vi "Main Page.vi"(8 "error in (no error)":errorcluster, 11 "Node Ptr":T2 format="%.0x") -> (0 "error out":errorcluster)   [LabVIEW 2019, in "Instrument Addon System Explorer.lvlib"]
uses:
  Instrument Addon System Explorer.lvlib
  <vilib>/NI VeriStand/Custom Device API/Custom Device Item Ref.ctl
  Addon Shared/Types/FG Control.ctl
  <vilib>/NI/NI VeriStand Hardware Resource Discovery/_Types/Filter Type.ctl
  Addon Shared/Constants.vi
  <vilib>/NI VeriStand/Custom Device API/NI VeriStand - Get Item Property.vi
  <vilib>/NI VeriStand/Custom Device API/Get Item Property (U32).vi
  <vilib>/NI VeriStand/Custom Device API/NI VeriStand - Set Item Property.vi
  <vilib>/NI VeriStand/Custom Device API/Set Item Property (U32).vi
  <vilib>/NI VeriStand/Custom Device API/Get Item Property (String).vi
  <vilib>/NI VeriStand/Custom Device API/Set Item Property (String).vi
  <vilib>/NI VeriStand/Custom Device API/Get Item Property (Boolean).vi
  <vilib>/NI VeriStand/Custom Device API/Set Item Property (Boolean).vi
  <vilib>/Utility/LVClass/Get LV Class Default Value.vi
  Support Libraries/Protocols/Protocols.lvlibp/Protocol Parent/Protocol Parent.lvclass
  <vilib>/NI VeriStand/Custom Device API/Custom Device API.lvlib
  Addon Shared/Instrument Addon Shared.lvlib
  <vilib>/NI/NI VeriStand Hardware Resource Discovery/NIVS Hardware Discovery.lvlib
panel:
  out "Version":string
  in  "PCL Decimation":u32=1 min=1 max=10000 step=1
  in  "Protocol Settings":enum32{"RS232", "VISA", "TCP/IP", "UDP"}(tab)=enum."VISA"
  in  "COM Browse":bool
  in  "Termination Character":u8=10 format="%.0x"
  in  "End Write":bool=TRUE caption="End Write on Termination Character?"
  in  "End Read":bool=TRUE caption="End Read on Termination Character?"
  in  "XOFF":T1(ring)=enum."DC3"
  in  "XON":T1(ring)=enum."DC1"
  in  "Flow Control":u16(ring) items=["None"=0, "XON/XOFF"=1, "RTS/CTS"=2, "DTR/DSR"=4]
  in  "Stop Bits":u16(ring)=10 items=["1.0"=10, "1.5"=15, "2.0"=20]
  in  "Parity":enum16{"None", "Odd", "Even", "Mark", "Space"}(ring)
  in  "Data Bits":u16=8 min=5 max=8 step=1
  in  "Baud Rate":u32(ring)=9600 items=["75"=75, "110"=110, "134"=134, "150"=150, "300"=300, "600"=600, "1200"=1200, "1800"=1800, "2400"=2400, "4800"=4800, "7200"=7200, "9600"=9600, "14400"=14400, "19200"=19200, "28800"=28800, "38400"=38400, "56000"=56000, "57600"=57600, "115200"=115200, "128000"=128000, "230400"=230400, "460800"=460800, "921600"=921600, "1843200"=1843200, "3000000"=3000000]
  in  "Port":string="COM1"
  in  "VISA Browse":bool
  in  "Append Write Termination Character":bool caption="End Write on Termination Character?"
  in  "Timeout":u32=2000 caption="Timeout (ms)"
  in  "Termination Character":u8=10 format="%.0x"
  in  "Enable Termination Character":bool=TRUE caption="Enable Termination Character?"
  in  "VISA Resource":string="GPIB0::2::INSTR"
  in  "Port":u16
  in  "IP Address":string="localhost"
  in  "UDP Browse":bool
  in  "Target Port":u16
  in  "Target IP Address":string="localhost"
  in  "Local Port":u16
  in  "Local IP Address":string="localhost"
  in  "Protocol":string(combo)
  in  "SHDocVw.IWebBrowser":refnum<k7>(container)
  in  "Header":cluster{"Section Name":string}={"Section Name"="Custom Device Item Settings"}
  in  "Description":string
  in  "Name":string
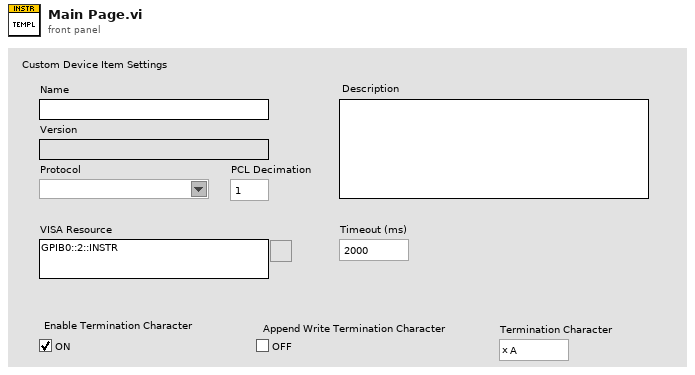
[diagram p1: front panel]
types:
  T1 = enum16{"NUL", "SOH", "STX", "ETX", "EOT", "ENQ", "ACK", "BEL", "BS", "HT", "LF", "VT", "FF", "CR", "SO", "SI", "DLE", "DC1", "DC2", "DC3", "DC4", "NAK", "SYN", "ETB", "CAN", "EM", "SUB", "ESC", "FS", "GS", "RS", "US", "SP", "!", "\"", "#", "$", "%", "&", "'", "(", ")", "*", "+", ",", "- (-)", ".", "/", "0", "1", "2", "3", "4", "5", "6", "7", "8", "9", ":", ";", "<", "=", ">", "?", "@", "A", "B", "C", "D", "E", "F", "G", "H", "I", "J", "K", "L", "M", "N", "O", "P", "Q", "R", "S", "T", "U", "V", "W", "X", "Y", "Z", "[", "\\", "]", "^", "_", "`", "a", "b", "c", "d", "e", "f", "g", "h", "i", "j", "k", "l", "m", "n", "o", "p", "q", "r", "s", "t", "u", "v", "w", "x", "y", "z", "{", "|", "}", "~"}
  T2 = typedef "Custom Device API.lvlib/Custom Device Item Ref.ctl" = u64
  T3 = typedef "Instrument Addon Shared.lvlib/FG Control.ctl" = enum16{"Get", "Set"}
  T4 = typedef "Custom Device API.lvlib/Custom Device Item Info.ctl" = cluster{"Name":string, "Is Channel":bool, "GUID":string, "Is Waveform":bool}
  T5 = typedef "NIVS Hardware Discovery.lvlib/Filter Type.ctl" = enum16{"Device Category", "Product Name", "Ethernet", "XNET", "VISA", "FPGA", "EtherCAT Master", "DAQmx", "GPIB", "Serial"}
  T6 = typedef "Custom Device API.lvlib/Custom Device Commands.ctl" = enum16{"Default", "Item renamed", "Shutdown", "Dynamic button pressed"}
  T7 = typedef "Instrument Addon Shared.lvlib/VISA Settings.ctl" = cluster{"VISA Resource":string, "Enable Termination Character":bool, "Termination Character":u8, "Timeout":u32, "Append Write Termination Character":bool}
  T8 = typedef "Instrument Addon Shared.lvlib/TCPIP Settings.ctl" = cluster{"IP Address":string, "Port":u16}
  T9 = typedef "Instrument Addon Shared.lvlib/UDP Settings.ctl" = cluster{"Local IP Address":string, "Local Port":u16, "Target IP Address":string, "Target Port":u16}
  T10 = typedef "Instrument Addon Shared.lvlib/RSXXX Port Settings.ctl" = cluster{"Port":string, "Baud Rate":u32, "Data Bits":u16, "Parity":enum16{"None", "Odd", "Even", "Mark", "Space"}, "Stop Bits":u16, "Flow Control":u16, "XON":enum16{"NUL", "SOH", "STX", "ETX", "EOT", "ENQ", "ACK", "BEL", "BS", "HT", "LF", "VT", "FF", "CR", "SO", "SI", "DLE", "DC1", "DC2", "DC3", "DC4", "NAK", "SYN", "ETB", "CAN", "EM", "SUB", "ESC", "FS", "GS", "RS", "US", "SP", "!", "\"", "#", "$", "%", "&", "'", "(", ")", "*", "+", ",", "- (-)", ".", "/", "0", "1", "2", "3", "4", "5", "6", "7", "8", "9", ":", ";", "<", "=", ">", "?", "@", "A", "B", "C", "D", "E", "F", "G", "H", "I", "J", "K", "L", "M", "N", "O", "P", "Q", "R", "S", "T", "U", "V", "W", "X", "Y", "Z", "[", "\\", "]", "^", "_", "`", "a", "b", "c", "d", "e", "f", "g", "h", "i", "j", "k", "l", "m", "n", "o", "p", "q", "r", "s", "t", "u", "v", "w", "x", "y", "z", "{", "|", "}", "~"}, "XOFF":enum16{"NUL", "SOH", "STX", "ETX", "EOT", "ENQ", "ACK", "BEL", "BS", "HT", "LF", "VT", "FF", "CR", "SO", "SI", "DLE", "DC1", "DC2", "DC3", "DC4", "NAK", "SYN", "ETB", "CAN", "EM", "SUB", "ESC", "FS", "GS", "RS", "US", "SP", "!", "\"", "#", "$", "%", "&", "'", "(", ")", "*", "+", ",", "- (-)", ".", "/", "0", "1", "2", "3", "4", "5", "6", "7", "8", "9", ":", ";", "<", "=", ">", "?", "@", "A", "B", "C", "D", "E", "F", "G", "H", "I", "J", "K", "L", "M", "N", "O", "P", "Q", "R", "S", "T", "U", "V", "W", "X", "Y", "Z", "[", "\\", "]", "^", "_", "`", "a", "b", "c", "d", "e", "f", "g", "h", "i", "j", "k", "l", "m", "n", "o", "p", "q", "r", "s", "t", "u", "v", "w", "x", "y", "z", "{", "|", "}", "~"}, "End Read on Termination Character":bool, "End Write on Termination Character":bool, "Termination Character":u8}
  T11 = typedef "Protocols.lvlibp/Protocol Parent.lvclass/Base Protocol Type.ctl" = enum16{"RS-XXX", "VISA", "TCPIP", "UDP"}
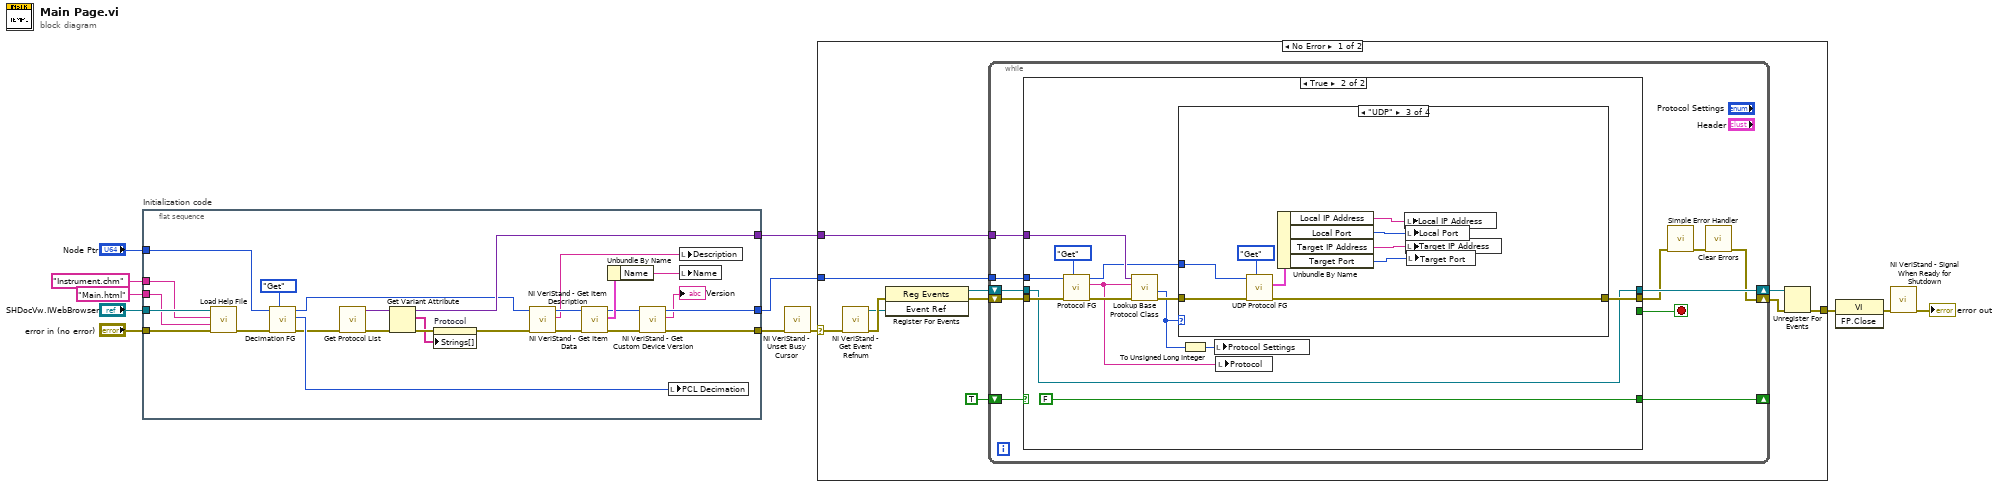
[diagram p0: block diagram]
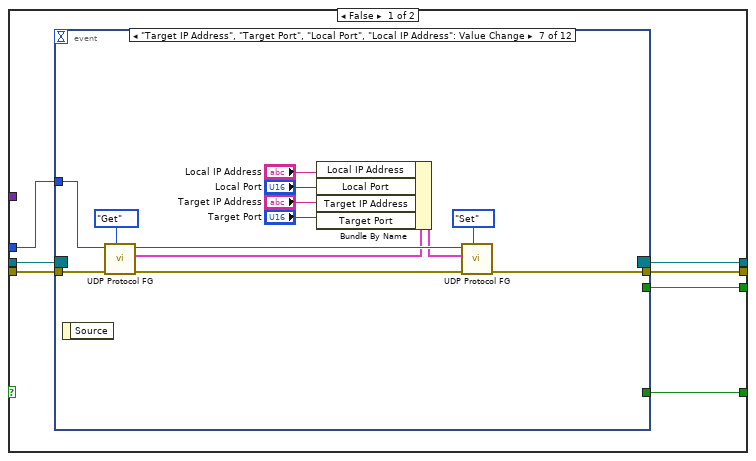
[diagram p2: hidden frame]
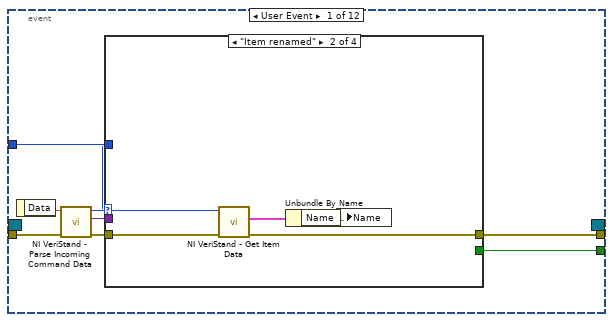
[diagram p3: hidden frame]
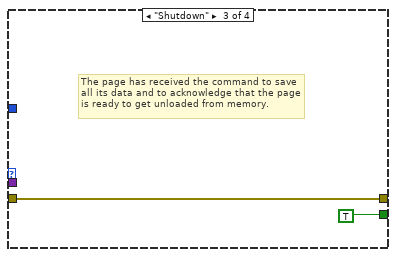
[diagram p5: hidden frame]
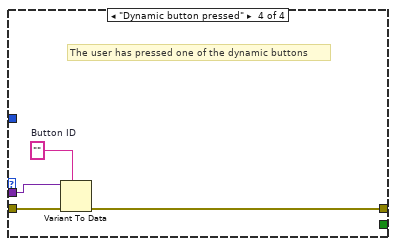
[diagram p6: hidden frame]
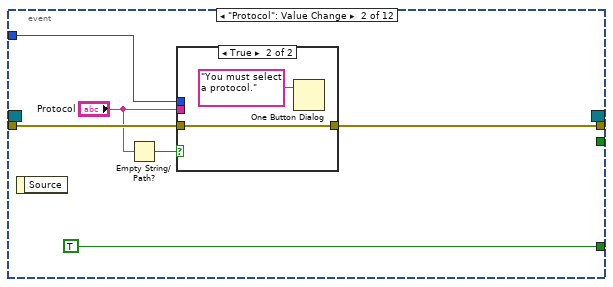
[diagram p7: hidden frame]
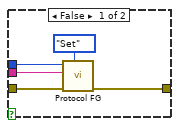
[diagram p8: hidden frame]
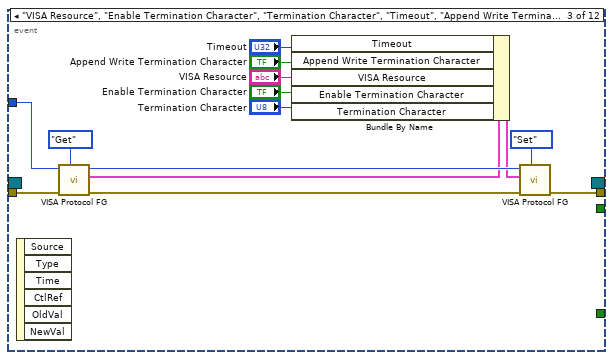
[diagram p9: hidden frame]
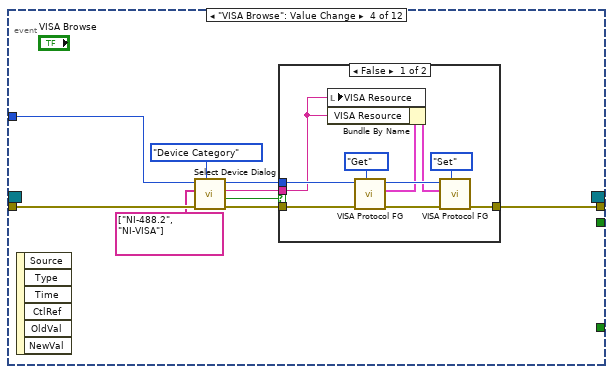
[diagram p10: hidden frame]
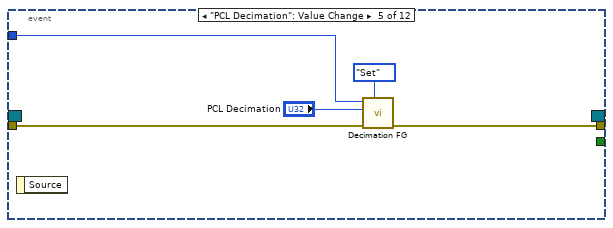
[diagram p12: hidden frame]
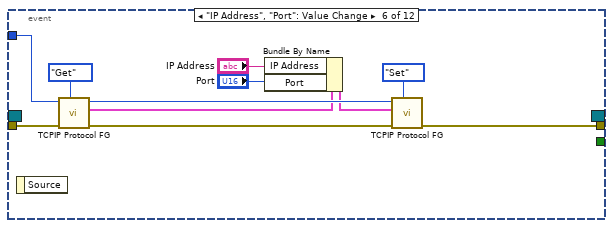
[diagram p13: hidden frame]
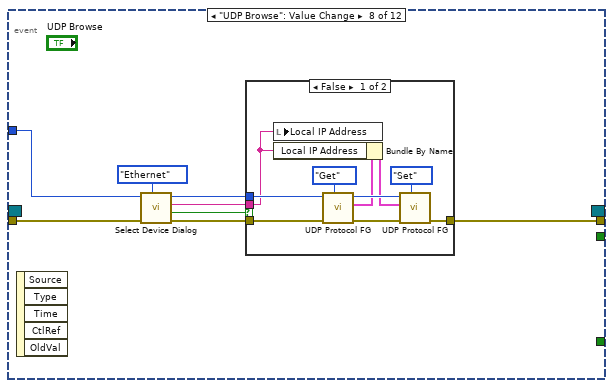
[diagram p14: hidden frame]
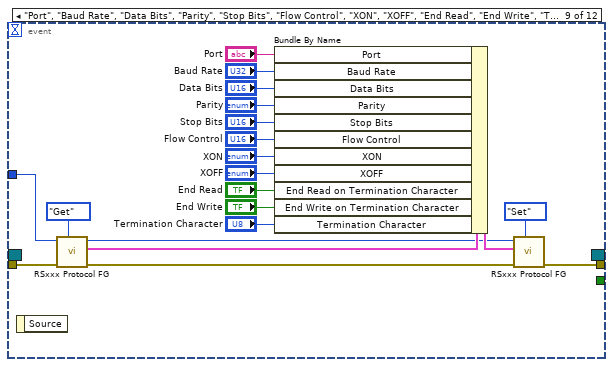
[diagram p16: hidden frame]
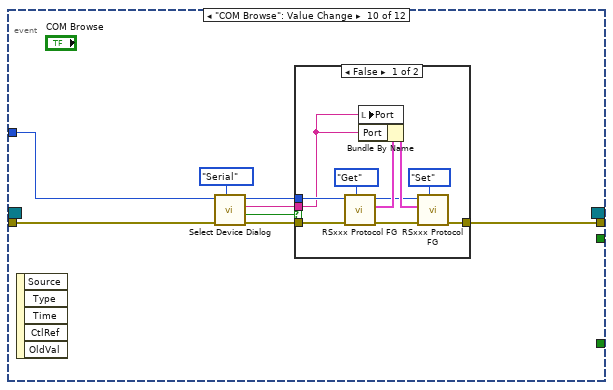
[diagram p17: hidden frame]
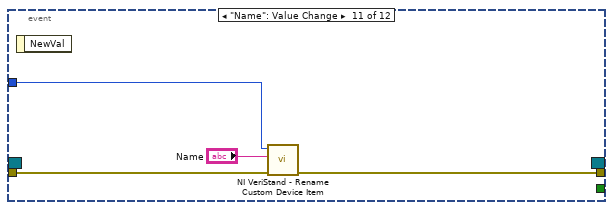
[diagram p19: hidden frame]
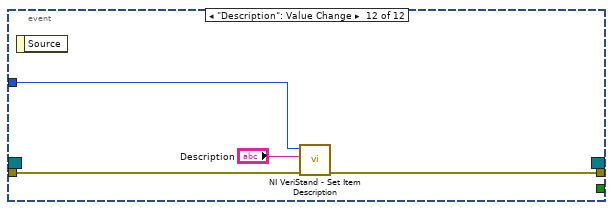
[diagram p20: hidden frame]
diagram:
  n1 = flat-sequence "Initialization code" {
    tunnel: "error in (no error)" -> [w33]
    tunnel: "Node Ptr" -> [w29]
    tunnel: [w16] -> w8
    tunnel: [w14] -> w5
    tunnel: "SHDocVw.IWebBrowser" -> [w32]
    tunnel: "Main.html" ("HTML File") -> [w31]
    tunnel: "Instrument.chm" ("Main CHM File") -> [w30]
    tunnel: [w21] -> w1
    frame #0 {
      n2 = call "Load Help File.vi"("error in (no error)"=w33, "HTML File"=w31, "Main CHM File"=w30, "SHDocVw.IWebBrowser2"=w32) -> ("error out"=w28:errorcluster)  [unwired: 7 in]
      n3 = call "Decimation FG.vi"("Action"=FG_Control."Get", "error in (no error)"=w28, "Device Item Ref in"=w29) -> ("error out"=w19:errorcluster, "Decimation out"=w26:u32, "Item Ref out"=w18:T2)  [unwired: 6 in]
      n4 = call "Get Protocol List.vi"("error in (no error)"=w19) -> ("error out"=w24:errorcluster, "Class Lookup"=w25:variant)  [unwired: 9 in]
      n5 = Get Variant Attribute(Variant=w25, error in=w24) -> (duplicate Variant=w21:variant, names=w22:string[], error out=w23:errorcluster)  [unwired: 2 in, 1 out]
      n6 = property on="Protocol" class="CmbBox"(error in=w23, "Strings[]"=w22) -> (error out=w20:errorcluster)  [unwired: 1 in, 1 out]
      n7 = call <vilib>:"NI VeriStand - Get Item Description.vi"("error in (no error)"=w20, "Item Ref in"=w18) -> ("error out"=w36:errorcluster, "Description"=w37:string, "Item Ref out"=w38:T2)  [unwired: 7 out]
      n8 = call <vilib>:"NI VeriStand - Get Item Data.vi"("error in (no error)"=w36, "Item Ref in"=w38) -> ("error out"=w17:errorcluster, "Item Info"=w35:T4, "Item Ref out"=w15:T2)  [unwired: 7 out]
      n9 = Unbundle By Name(w35) -> ("Name"=w34:string)
      n10 = call <vilib>:"NI VeriStand - Get Custom Device Version.vi"("error in (no error)"=w17, "Device Ref in"=w15) -> ("error out"=w16:errorcluster, "Value"=→"Version":string, "Device Ref out"=w14:T2)  [unwired: 7 in]
      n11 = local write "PCL Decimation"(w26) -> ()
      n12 = local write "Description"(w37) -> ()
      n13 = local write "Name"(w34) -> ()
    }
  }
  n14 = call <vilib>:"NI VeriStand - Unset Busy Cursor.vi"("error in (no error)"=w8) -> ("error out"=w7:errorcluster)  [unwired: 10 out]
  n15 = case shown="No Error" w7 {
    selector: w7 -> [w41 w287]
    tunnel: [w46 w285] -> w12
    tunnel: w5 -> [w42 _]
    tunnel: w1 -> [w40 _]
    frame No Error {
      n16 = call <vilib>:"NI VeriStand - Get Event Refnum.vi"("error in (no error)"=w41) -> ("error out"=w49:errorcluster, "Event Ref"=w45:refnum<user-event>)  [unwired: 9 out]
      n17 = register-events(error in=w49, w45) -> (reference out=w43:refnum<event-registration>, error out=w44:errorcluster)  [unwired: 1 in]
      n18 = while {
        tunnel: w42 -> [w56]
        shift-right: [w53] -> w47
        shift-left: w44 -> [w59]
        shift-right: [w60] -> w48
        shift-left: w43 -> [w58]
        tunnel: w40 -> [w52]
        shift-right: [w50] -> _
        shift-left: TRUE -> [w51]
        stop <- w57 stop-if-true
        n19 = case shown="True" w51 {
          tunnel: [w67 w232] -> w60
          tunnel: w59 -> [w66 w241]
          tunnel: w58 -> [w65 w232]
          tunnel: [w64 _] -> w57
          tunnel: w56 -> [w63 w240]
          tunnel: [w62 w233] -> w55
          tunnel: w52 -> [_ w238]
          tunnel: [w61 FALSE] -> w50
          frame False {
            n20 = event shown="[6] \"Target IP Address\", \"Target Port\", \"Local Port\", \"Local IP Address\": Value Change" {
              selector: w65 -> [_ _ _ _ _ _ _ _ _ _ _ _]
              dyn-events: [_ _ _ _ _ _ _ _ _ _ _ _] -> w67
              timeout: _ -> [_ _ _ _ _ _ _ _ _ _ _ _]
              tunnel: w66 -> [w75 w92 w113 w122 w138 w149 w162 w170 w199 w209 w225 w228]
              tunnel: [w71 _ _ _ _ _ _ _ _ _ _ _] -> w64
              tunnel: [w70 w88 w109 w123 w136 w145 w158 w171 w201 w210 w224 w227] -> w62
              tunnel: w63 -> [w69 w93 w112 w120 w137 w148 w161 w168 w197 w208 w223 w229]
              tunnel: [_ TRUE _ _ _ _ _ _ _ _ _ _] -> w61
              event User Event {
                n21 = event-data() -> ("Data"=w74:string)  [unwired: 1 out]
                n22 = call <vilib>:"NI VeriStand - Parse Incoming Command Data.vi"("error in (no error)"=w75, "Incoming data"=w74) -> ("error out"=w73:errorcluster, "Outgoing data"=w68:variant, "Action"=w72:T6)  [unwired: 7 out]
                n23 = case shown="\"Item renamed\"" w72 {
                  tunnel: w73 -> [w76 w81 w82 w87]
                  tunnel: [_ _ TRUE _] -> w71
                  tunnel: [w76 w78 w82 w84] -> w70
                  tunnel: w69 -> [_ w80 _ _]
                  tunnel: w68 -> [_ _ _ w86]
                  frame "Default", Default {
                  }
                  frame "Item renamed" {
                    n24 = call <vilib>:"NI VeriStand - Get Item Data.vi"("error in (no error)"=w81, "Item Ref in"=w80) -> ("error out"=w78:errorcluster, "Item Info"=w79:T4)  [unwired: 8 out]
                    n25 = Unbundle By Name(w79) -> ("Name"=w77:string)
                    n26 = local write "Name"(w77) -> ()
                  }
                  frame "Shutdown" {
                    # "The page has received the command to save all its data and to acknowledge that the page is ready to get unloaded from memory."
                  }
                  frame "Dynamic button pressed" {
                    w85 = ""  # Button ID
                    # "The user has pressed one of the dynamic buttons"
                    n27 = Variant To Data(error in=w87, type=w85, Variant=w86) -> (error out=w84:errorcluster)  [unwired: 1 out]
                  }
                }
              }
              event "Protocol": Value Change {
                n28 = event-data() -> ()  [unwired: 2 out]
                n29 = Empty String/Path?(string/path="Protocol") -> (empty?=w90:bool)
                n30 = case shown="True" w90 {
                  tunnel: w93 -> [w96 _]
                  tunnel: w92 -> [w97 w99]
                  tunnel: [w94 w99] -> w88
                  tunnel: "Protocol" -> [w95 _]
                  frame False {
                    n31 = call "Protocol FG.vi"("Action"=FG_Control."Set", "error in (no error)"=w97, "Protocol"=w95, "Device Item Ref in"=w96) -> ("error out"=w94:errorcluster)  [unwired: 5 in, 2 out]
                  }
                  frame True {
                    n32 = One Button Dialog(message="You must select a protocol.") -> ()  [unwired: 1 in, 1 out]
                  }
                }
              }
              event "VISA Resource", "Enable Termination Character", "Termination Character", "Timeout", "Append Write Termination Character": Value Change {
                n33 = event-data() -> ()  [unwired: 7 out]
                n34 = call "VISA Protocol FG.vi"("Action"=FG_Control."Get", "error in (no error)"=w113, "Device Item Ref in"=w112) -> ("error out"=w110:errorcluster, "VISA Config"=w107:T7, "Item Ref out"=w108:T2)  [unwired: 6 in]
                n35 = Bundle By Name(cluster=w107, "Timeout"="Timeout", "Append Write Termination Character"="Append Write Termination Character", "VISA Resource"="VISA Resource", "Enable Termination Character"="Enable Termination Character", "Termination Character"="Termination Character") -> (w106:T7)
                n36 = call "VISA Protocol FG.vi"("Action"=FG_Control."Set", "error in (no error)"=w110, "VISA Config"=w106, "Device Item Ref in"=w108) -> ("error out"=w109:errorcluster)  [unwired: 5 in, 2 out]
              }
              event "VISA Browse": Value Change {
                n37 = event-data() -> ()  [unwired: 7 out]
                n38 = call <vilib>:"Select Device Dialog.vi"("Filter Type"=Filter_Type."Device Category", "error in (no error)"=w122, "Filter Names"=string[] ["NI-488.2", "NI-VISA"], "Item Ref in"=w120) -> ("error out"=w121:errorcluster, "Cancelled?"=w118:bool, "Selected Alias"=w117:string, "Item Ref out"=w119:T2)  [unwired: 4 in]
                n39 = case shown="False" w118 {
                  tunnel: w121 -> [w132 w134]
                  tunnel: w119 -> [w131 _]
                  tunnel: [w128 w134] -> w123
                  tunnel: w117 -> [w124 _]
                  frame False {
                    n40 = local write "VISA Resource"(w124) -> ()
                    n41 = call "VISA Protocol FG.vi"("Action"=FG_Control."Get", "error in (no error)"=w132, "Device Item Ref in"=w131) -> ("error out"=w129:errorcluster, "VISA Config"=w126:T7, "Item Ref out"=w127:T2)  [unwired: 6 in]
                    n42 = Bundle By Name(cluster=w126, "VISA Resource"=w124) -> (w125:T7)
                    n43 = call "VISA Protocol FG.vi"("Action"=FG_Control."Set", "error in (no error)"=w129, "VISA Config"=w125, "Device Item Ref in"=w127) -> ("error out"=w128:errorcluster)  [unwired: 5 in, 2 out]
                  }
                  frame True {
                  }
                }
              }
              event "PCL Decimation": Value Change {
                n44 = event-data() -> ()  [unwired: 2 out]
                n45 = call "Decimation FG.vi"("Action"=FG_Control."Set", "error in (no error)"=w138, "Decimation"="PCL Decimation", "Device Item Ref in"=w137) -> ("error out"=w136:errorcluster)  [unwired: 5 in, 2 out]
              }
              event "IP Address", "Port": Value Change {
                n46 = event-data() -> ()  [unwired: 2 out]
                n47 = call "TCPIP Protocol FG.vi"("Action"=FG_Control."Get", "error in (no error)"=w149, "Device Item Ref in"=w148) -> ("error out"=w146:errorcluster, "TCP/IP Config"=w143:T8, "Item Ref out"=w144:T2)  [unwired: 6 in]
                n48 = Bundle By Name(cluster=w143, "IP Address"="IP Address", "Port"="Port") -> (w142:T8)
                n49 = call "TCPIP Protocol FG.vi"("Action"=FG_Control."Set", "error in (no error)"=w146, "TCP/IP Config"=w142, "Device Item Ref in"=w144) -> ("error out"=w145:errorcluster)  [unwired: 5 in, 2 out]
              }
              event "Target IP Address", "Target Port", "Local Port", "Local IP Address": Value Change {
                n50 = event-data() -> ()  [unwired: 2 out]
                n51 = call "UDP Protocol FG.vi"("Action"=FG_Control."Get", "error in (no error)"=w162, "Device Item Ref in"=w161) -> ("error out"=w159:errorcluster, "UDP Config"=w156:T9, "Item Ref out"=w157:T2)  [unwired: 6 in]
                n52 = Bundle By Name(cluster=w156, "Local IP Address"="Local IP Address", "Local Port"="Local Port", "Target IP Address"="Target IP Address", "Target Port"="Target Port") -> (w155:T9)
                n53 = call "UDP Protocol FG.vi"("Action"=FG_Control."Set", "error in (no error)"=w159, "UDP Config"=w155, "Device Item Ref in"=w157) -> ("error out"=w158:errorcluster)  [unwired: 5 in, 2 out]
              }
              event "UDP Browse": Value Change {
                n54 = event-data() -> ()  [unwired: 6 out]
                n55 = call <vilib>:"Select Device Dialog.vi"("Filter Type"=Filter_Type."Ethernet", "error in (no error)"=w170, "Item Ref in"=w168) -> ("error out"=w169:errorcluster, "Cancelled?"=w166:bool, "Selected Alias"=w165:string, "Item Ref out"=w167:T2)  [unwired: 5 in]
                n56 = case shown="False" w166 {
                  tunnel: w169 -> [w180 w182]
                  tunnel: w167 -> [w179 _]
                  tunnel: [w176 w182] -> w171
                  tunnel: w165 -> [w172 _]
                  frame False {
                    n57 = local write "Local IP Address"(w172) -> ()
                    n58 = call "UDP Protocol FG.vi"("Action"=FG_Control."Get", "error in (no error)"=w180, "Device Item Ref in"=w179) -> ("error out"=w177:errorcluster, "UDP Config"=w174:T9, "Item Ref out"=w175:T2)  [unwired: 6 in]
                    n59 = Bundle By Name(cluster=w174, "Local IP Address"=w172) -> (w173:T9)
                    n60 = call "UDP Protocol FG.vi"("Action"=FG_Control."Set", "error in (no error)"=w177, "UDP Config"=w173, "Device Item Ref in"=w175) -> ("error out"=w176:errorcluster)  [unwired: 5 in, 2 out]
                  }
                  frame True {
                  }
                }
              }
              event "Port", "Baud Rate", "Data Bits", "Parity", "Stop Bits", "Flow Control", "XON", "XOFF", "End Read", "End Write", "Termination Character": Value Change {
                n61 = event-data() -> ()  [unwired: 2 out]
                n62 = call "RSxxx Protocol FG.vi"("Action"=FG_Control."Get", "error in (no error)"=w199, "Device Item Ref in"=w197) -> ("error out"=w198:errorcluster, "Serial Config"=w196:T10, "Item Ref out"=w183:T2)  [unwired: 6 in]
                n63 = Bundle By Name(cluster=w196, "Port"="Port", "Baud Rate"="Baud Rate", "Data Bits"="Data Bits", "Parity"="Parity", "Stop Bits"="Stop Bits", "Flow Control"="Flow Control", "XON"="XON", "XOFF"="XOFF", "End Read on Termination Character"="End Read", "End Write on Termination Character"="End Write", "Termination Character"="Termination Character") -> (w195:T10)
                n64 = call "RSxxx Protocol FG.vi"("Action"=FG_Control."Set", "error in (no error)"=w198, "Serial Config"=w195, "Device Item Ref in"=w183) -> ("error out"=w201:errorcluster)  [unwired: 5 in, 2 out]
              }
              event "COM Browse": Value Change {
                n65 = event-data() -> ()  [unwired: 6 out]
                n66 = call <vilib>:"Select Device Dialog.vi"("Filter Type"=Filter_Type."Serial", "error in (no error)"=w209, "Item Ref in"=w208) -> ("error out"=w206:errorcluster, "Cancelled?"=w205:bool, "Selected Alias"=w204:string, "Item Ref out"=w207:T2)  [unwired: 5 in]
                n67 = case shown="False" w205 {
                  tunnel: [w219 w221] -> w210
                  tunnel: w206 -> [w217 w221]
                  tunnel: w207 -> [w215 _]
                  tunnel: w204 -> [w211 _]
                  frame False {
                    n68 = call "RSxxx Protocol FG.vi"("Action"=FG_Control."Get", "error in (no error)"=w217, "Device Item Ref in"=w215) -> ("error out"=w216:errorcluster, "Serial Config"=w214:T10, "Item Ref out"=w212:T2)  [unwired: 6 in]
                    n69 = local write "Port"(w211) -> ()
                    n70 = Bundle By Name(cluster=w214, "Port"=w211) -> (w213:T10)
                    n71 = call "RSxxx Protocol FG.vi"("Action"=FG_Control."Set", "error in (no error)"=w216, "Serial Config"=w213, "Device Item Ref in"=w212) -> ("error out"=w219:errorcluster)  [unwired: 5 in, 2 out]
                  }
                  frame True {
                  }
                }
              }
              event "Name": Value Change {
                n72 = event-data() -> ()  [unwired: 2 out]
                n73 = call <vilib>:"NI VeriStand - Rename Custom Device Item.vi"("error in (no error)"=w225, "New Name"="Name", "Item Ref in"=w223) -> ("error out"=w224:errorcluster)  [unwired: 1 in, 7 out]
              }
              event "Description": Value Change {
                n74 = event-data() -> ()  [unwired: 2 out]
                n75 = call <vilib>:"NI VeriStand - Set Item Description.vi"("error in (no error)"=w228, "Description"="Description", "Item Ref in"=w229) -> ("error out"=w227:errorcluster)  [unwired: 8 out]
              }
            }
          }
          frame True {
            n76 = call "Protocol FG.vi"("Action"=FG_Control."Get", "error in (no error)"=w241, "Device Item Ref in"=w240) -> ("error out"=w237:errorcluster, "Protocol out"=w234:string, "Item Ref out"=w236:T2)  [unwired: 6 in]
            n77 = call "Lookup Base Protocol Class.vi"("error in (no error)"=w237, "Protocol in"=w234, "Class Lookup"=w238) -> ("error out"=w239:errorcluster, "Protocol out"=w231:T11)  [unwired: 5 in, 2 out]
            n78 = case shown="\"UDP\"" w231 {
              tunnel: w239 -> [w252 w259 w268 w284]
              tunnel: [w251 w258 w267 w283] -> w233
              tunnel: w236 -> [w250 w257 w266 w282]
              frame "VISA" {
                n79 = call "VISA Protocol FG.vi"("Action"=FG_Control."Get", "error in (no error)"=w252, "Device Item Ref in"=w250) -> ("error out"=w251:errorcluster, "VISA Config"=w248:T7)  [unwired: 6 in, 1 out]
                n80 = Unbundle By Name(w248) -> ("Append Write Termination Character"=w243:bool, "Timeout"=w244:u32, "VISA Resource"=w247:string, "Enable Termination Character"=w246:bool, "Termination Character"=w245:u8)
                n81 = local write "Append Write Termination Character"(w243) -> ()
                n82 = local write "Enable Termination Character"(w246) -> ()
                n83 = local write "Termination Character"(w245) -> ()
                n84 = local write "Timeout"(w244) -> ()
                n85 = local write "VISA Resource"(w247) -> ()
              }
              frame "TCPIP" {
                n86 = call "TCPIP Protocol FG.vi"("Action"=FG_Control."Get", "error in (no error)"=w259, "Device Item Ref in"=w257) -> ("error out"=w258:errorcluster, "TCP/IP Config"=w255:T8)  [unwired: 6 in, 1 out]
                n87 = Unbundle By Name(w255) -> ("IP Address"=w254:string, "Port"=w253:u16)
                n88 = local write "IP Address"(w254) -> ()
                n89 = local write "Port"(w253) -> ()
              }
              frame "UDP" {
                n90 = call "UDP Protocol FG.vi"("Action"=FG_Control."Get", "error in (no error)"=w268, "Device Item Ref in"=w266) -> ("error out"=w267:errorcluster, "UDP Config"=w264:T9)  [unwired: 6 in, 1 out]
                n91 = Unbundle By Name(w264) -> ("Local IP Address"=w263:string, "Local Port"=w262:u16, "Target IP Address"=w261:string, "Target Port"=w260:u16)
                n92 = local write "Local IP Address"(w263) -> ()
                n93 = local write "Local Port"(w262) -> ()
                n94 = local write "Target IP Address"(w261) -> ()
                n95 = local write "Target Port"(w260) -> ()
              }
              frame "RS-XXX" {
                n96 = call "RSxxx Protocol FG.vi"("Action"=FG_Control."Get", "error in (no error)"=w284, "Device Item Ref in"=w282) -> ("error out"=w283:errorcluster, "Serial Config"=w280:T10)  [unwired: 6 in, 1 out]
                n97 = Unbundle By Name(w280) -> ("Port"=w279:string, "Baud Rate"=w278:u32, "Data Bits"=w269:u16, "Parity"=w270:enum16{"None", "Odd", "Even", "Mark", "Space"}, "Stop Bits"=w271:u16, "Flow Control"=w272:u16, "XON"=w273:T1, "XOFF"=w274:T1, "End Read on Termination Character"=w275:bool, "End Write on Termination Character"=w276:bool, "Termination Character"=w277:u8)
                n98 = local write "Termination Character"(w277) -> ()
                n99 = local write "Flow Control"(w272) -> ()
                n100 = local write "Data Bits"(w269) -> ()
                n101 = local write "Stop Bits"(w271) -> ()
                n102 = local write "XON"(w273) -> ()
                n103 = local write "End Write"(w276) -> ()
                n104 = local write "Port"(w279) -> ()
                n105 = local write "Baud Rate"(w278) -> ()
                n106 = local write "Parity"(w270) -> ()
                n107 = local write "XOFF"(w274) -> ()
                n108 = local write "End Read"(w275) -> ()
              }
            }
            n109 = To Unsigned Long Integer(number=w231) -> (unsigned 32bit integer=w235:u32)
            n110 = local write "Protocol Settings"(w235) -> ()
            n111 = local write "Protocol"(w234) -> ()
          }
        }
        n112 = call <vilib>:"Simple Error Handler.vi"("error in (no error)"=w55) -> ("error out"=w54:errorcluster)  [unwired: 1 in, 7 out]
        n113 = call <vilib>:"Clear Errors.vi"("error in (no error)"=w54) -> ("error out"=w53:errorcluster)  [unwired: 1 in, 5 out]
      }
      n114 = Unregister For Events(event registration refnum=w48, error in=w47) -> (error out=w46:errorcluster)
    }
    frame Error {
      n115 = call <vilib>:"Simple Error Handler.vi"("error in (no error)"=w287) -> ("error out"=w286:errorcluster)  [unwired: 1 in, 7 out]
      n116 = call <vilib>:"Clear Errors.vi"("error in (no error)"=w286) -> ("error out"=w285:errorcluster)  [unwired: 1 in, 5 out]
    }
  }
  n117 = invoke class="VI" method="FP.Close"(error in=w12) -> (error out=w11:errorcluster)  [unwired: 2 in, 2 out]
  n118 = call <vilib>:"NI VeriStand - Signal When Ready for Shutdown.vi"("error in (no error)"=w11) -> ("error out"=→"error out":errorcluster)  [unwired: 10 out]
